vi "configure runtime data.vi"(4 "output dictionary":refnum<class "data dictionary.lvclass">, 6 "input dictionary":refnum<class "data dictionary.lvclass">, 8 "error in":errorcluster, 10 "Slave Info List":T4(array[cluster]), 11 "Profibus Module configuration in":refnum<class "Profibus Module configuration.lvclass">) -> (0 "error out":errorcluster, 2 "inputs":T1[](array[typedef]), 3 "outputs":T1[](array[typedef]))   [LabVIEW 2013, in "Profibus Module runtime.lvclass"]
uses:
  Profibus Module runtime.lvclass
  configuration/Profibus Module configuration.lvclass
  profibus slave configuration.ctl
  profibus mapping configuration.ctl
  <vilib>/NI/Tag Bus/tag/Data Type.ctl
  <vilib>/NI/Tag Bus/dictionary/data dictionary.lvclass
  configuration/Profibus Module configuration.lvclass/Profibus Module configuration.ctl
  channel/Profibus channel.lvclass/Profibus channel.ctl
  <vilib>/NI/Tag Bus Module Framework/channel/TBM channel.lvclass/TBM channel.ctl
  <vilib>/NI/Tag Bus/tag/tag descriptor.lvclass/tag descriptor.ctl
  <vilib>/NI/Tag Bus/tag/tag descriptor.lvclass
  <vilib>/NI/Tag Bus Module Framework/channel/TBM channel.lvclass
  channel/Profibus channel.lvclass
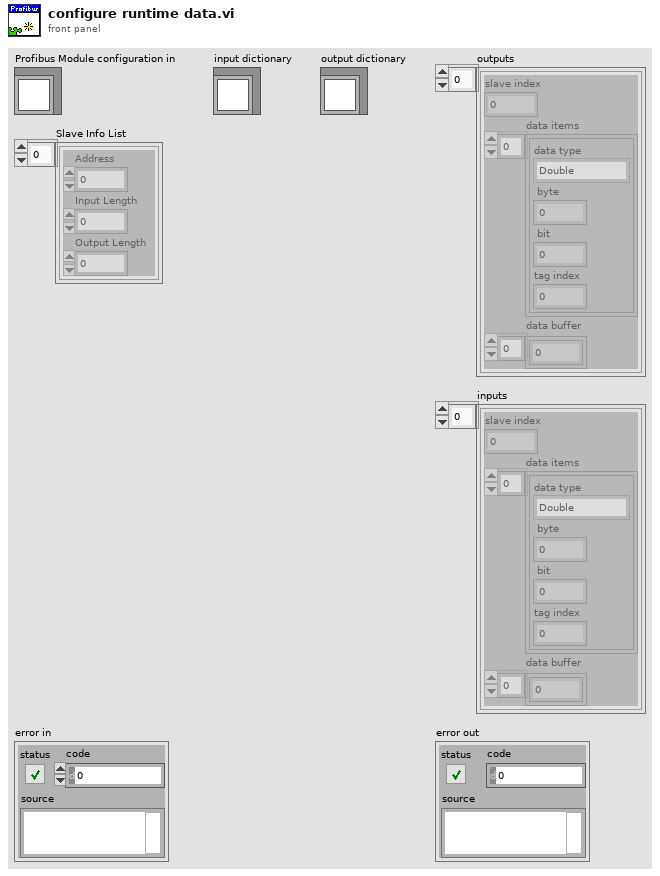
[diagram p1: front panel]
types:
  T1 = typedef "Profibus Module runtime.lvclass/profibus slave configuration.ctl" = cluster{"slave index":i8, "data items":T2[], "data buffer":u8[]}
  T2 = typedef "Profibus Module runtime.lvclass/profibus mapping configuration.ctl" = cluster{"data type":T3, " byte":i32, " bit":i32, "tag index":i32}
  T3 = typedef "tag bus.lvlib/tag descriptor.lvclass/Data Type.ctl" = enum16{"Double", "Single", "I64", "I32", "I16", "I8", "U64", "U32", "U16", "U8", "Boolean", "String", "Array of Double", "Array of Single", "Array of I64", "Array of I32", "Array of I16", "Array of I8", "Array of U64", "Array of U32", "Array of U16", "Array of U8", "Array of Boolean", "Array of String"}
  T4 = cluster{"Address":i8, "Input Length":u8, "Output Length":u8}[]
  T5 = typedef "TBM channel.lvclass/channel classification.ctl" = enum16{"input data", "output data", "processing parameter", "processing result"}
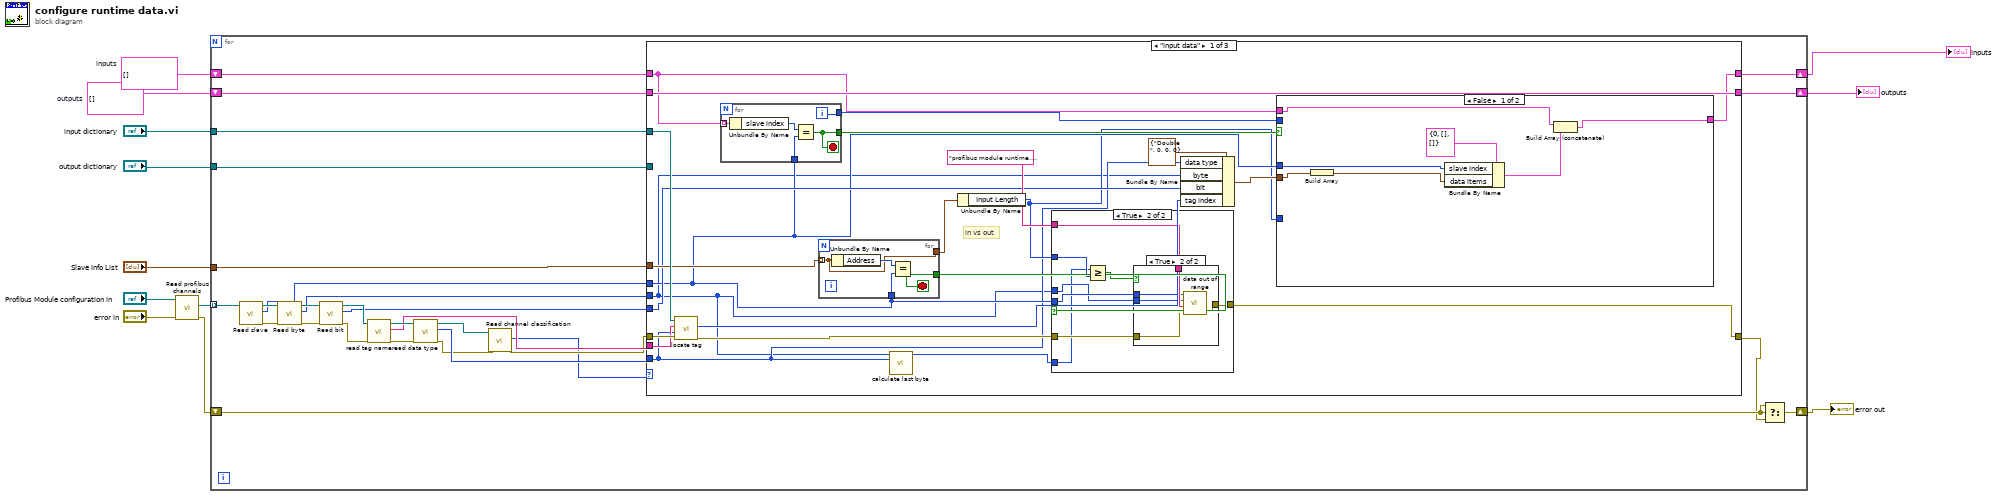
[diagram p0: block diagram]
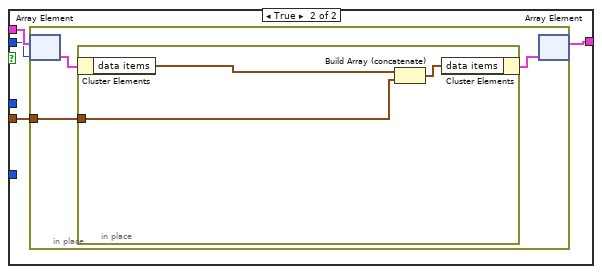
[diagram p2: hidden frame]
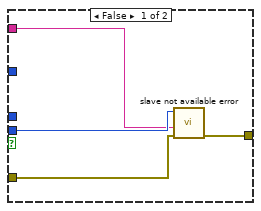
[diagram p3: hidden frame]
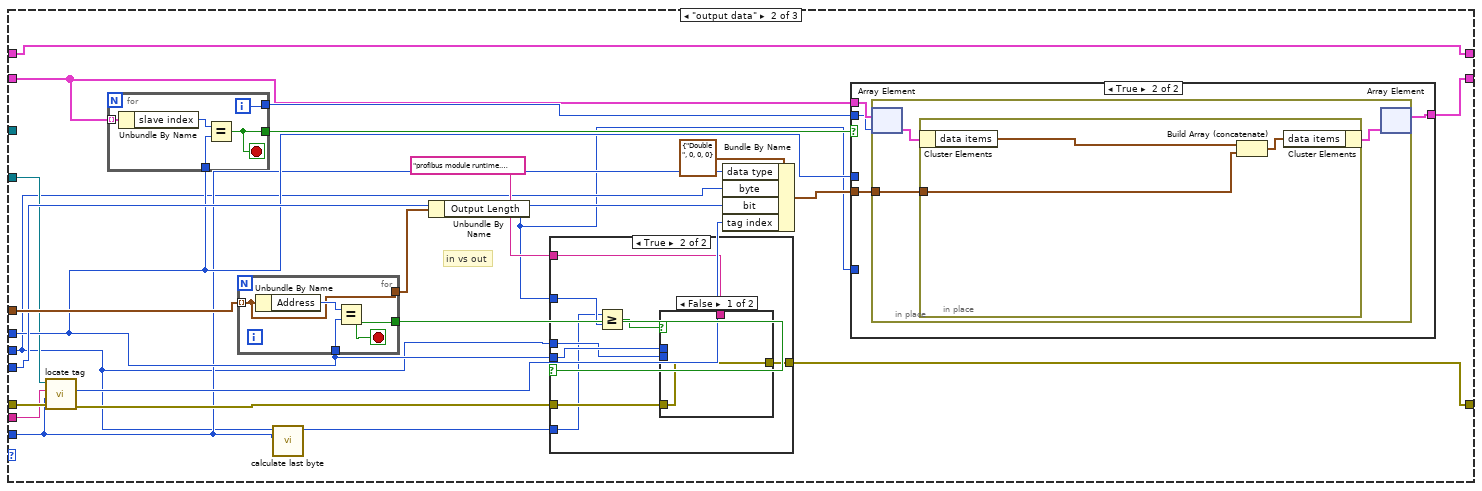
[diagram p5: hidden frame]
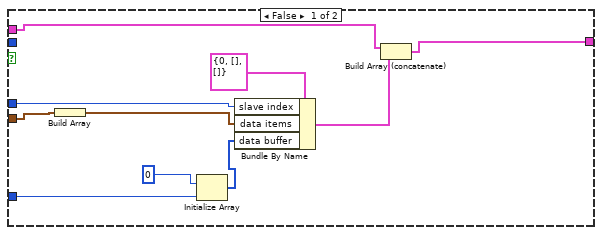
[diagram p6: hidden frame]
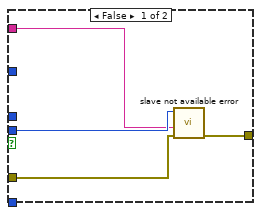
[diagram p7: hidden frame]
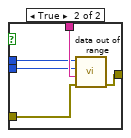
[diagram p8: hidden frame]
diagram:
  w6 = T1[] []  # outputs
  w7 = T1[] []  # inputs
  n1 = call "Read profibus channels.vi"("error in"="error in", "Profibus Module configuration in"="Profibus Module configuration in") -> ("error out"=w10:errorcluster, "channels"=w8:refnum<class "Profibus channel.lvclass">[])  [unwired: 7 in, 1 out]
  n2 = for {
    shift-right: [w39] -> w9
    shift-left: w10 -> [w40]
    tunnel: w8 -> [w22] mode=indexing
    shift-right: [w35] -> w1
    shift-left: w7 -> [w34]
    shift-right: [w33] -> w5
    shift-left: w6 -> [w32]
    tunnel: "Slave Info List" -> [w36]
    tunnel: "input dictionary" -> [w38]
    tunnel: "output dictionary" -> [w37]
    n3 = call "Read slave.vi"("Profibus channel in"=w22) -> ("error out"=w19:errorcluster, "slave"=w15:i8, "Profibus channel out"=w20:refnum<class "Profibus channel.lvclass">)  [unwired: 8 in]
    n4 = call "Read byte.vi"("error in"=w19, "Profibus channel in"=w20) -> ("error out"=w18:errorcluster, "byte"=w14:i32, "Profibus channel out"=w21:refnum<class "Profibus channel.lvclass">)  [unwired: 7 in]
    n5 = call "Read bit.vi"("error in"=w18, "Profibus channel in"=w21) -> ("error out"=w17:errorcluster, "bit"=w13:i32, "Profibus channel out"=w16:refnum<class "Profibus channel.lvclass">)  [unwired: 7 in]
    n6 = call <vilib>:"read tag name.vi"("error in"=w17, "system tag in"=w16) -> ("error out"=w27:errorcluster, "name"=w28:string, "system tag out"=w30:refnum<class "Profibus channel.lvclass">)  [unwired: 7 in]
    n7 = call <vilib>:"read data type.vi"("error in"=w27, "system tag in"=w30) -> ("error out"=w25:errorcluster, "data type"=w26:T3, "system tag out"=w29:refnum<class "Profibus channel.lvclass">)  [unwired: 7 in]
    n8 = call <vilib>:"Read channel classification.vi"("error in"=w25, "channel in"=w29) -> ("error out"=w24:errorcluster, "channel classification"=w23:T5)  [unwired: 7 in, 1 out]
    n9 = case shown="\"input data\"" w23 {
      tunnel: w24 -> [w62 w130 w178]
      tunnel: w26 -> [w43 w111 _]
      tunnel: w38 -> [w60 _ _]
      tunnel: w37 -> [_ w115 _]
      tunnel: w36 -> [w59 w128 _]
      tunnel: [w50 w112 w180] -> w35
      tunnel: w34 -> [w51 w112 w180]
      tunnel: [w63 w113 w179] -> w33
      tunnel: w32 -> [w63 w114 w179]
      tunnel: [w57 w126 w178] -> w31
      tunnel: w15 -> [w45 w116 _]
      tunnel: w14 -> [w42 w110 _]
      tunnel: w13 -> [w47 w118 _]
      tunnel: w28 -> [w61 w129 _]
      frame "input data" {
        # "in vs out"
        n10 = call <vilib>:"locate tag.vi"("error in"=w62, "data type"=w43, "name"=w61, "data dictionary in"=w60) -> ("error out"=w58:errorcluster, "index"=w46:i32)  [unwired: 5 in, 1 out]
        n11 = for {
          tunnel: w51 -> [w107] mode=indexing
          tunnel: w45 -> [w105]
          tunnel: [w104] -> w53
          tunnel: [w103] -> w52
          i -> [w103]
          stop <- w104 stop-if-true
          n12 = Unbundle By Name(w107) -> ("slave index"=w106:i8)
          n13 = Equal?(x=w106, y=w105) -> (x = y?=w104:bool)
        }
        n14 = for {
          tunnel: w59 -> [w99] mode=indexing
          tunnel: w45 -> [w101]
          tunnel: [w100] -> w56
          tunnel: [w99] -> w55
          stop <- w100 stop-if-true
          n15 = Unbundle By Name(w99) -> ("Address"=w102:i8)
          n16 = Equal?(x=w102, y=w101) -> (x = y?=w100:bool)
        }
        n17 = call "calculate last byte.vi"("type"=w43, "byte in"=w42) -> ("last byte"=w41:i32)  [unwired: 9 in]
        n18 = Unbundle By Name(w55) -> ("Input Length"=w44:u8)
        n19 = case shown="True" w56 {
          tunnel: w58 -> [w84 w91]
          tunnel: [w83 w92] -> w57
          tunnel: w45 -> [w82 w88]
          tunnel: w44 -> [_ w89]
          tunnel: w42 -> [_ w87]
          tunnel: "profibus module runtime.lvclass>>init.vi>>configure runtime data.vi" ("source") -> [w81 w90]
          tunnel: w41 -> [_ w85]
          frame False {
            n20 = call "slave not available error.vi"("error in"=w84, "source"=w81, "slave"=w82) -> ("error out"=w83:errorcluster)  [unwired: 8 in]
          }
          frame True {
            n21 = Greater Or Equal?(x=w85, y=w89) -> (x >= y?=w86:bool)
            n22 = case shown="True" w86 {
              tunnel: [w93 w98] -> w92
              tunnel: w91 -> [w93 w97]
              tunnel: w90 -> [_ w96]
              tunnel: w88 -> [_ w95]
              tunnel: w87 -> [_ w94]
              frame False {
              }
              frame True {
                n23 = call "data out of range.vi"("error in"=w97, "source"=w96, "byte"=w94, "slave"=w95) -> ("error out"=w98:errorcluster)  [unwired: 7 in]
              }
            }
          }
        }
        n24 = Bundle By Name(cluster=T2 {"data type"=enum."Double", " byte"=0, " bit"=0, "tag index"=0} ("data items"), "data type"=w43, "byte"=w42, "bit"=w47, "tag index"=w46) -> (w48:T2)
        n25 = case shown="False" w53 {
          tunnel: w52 -> [_ w73]
          tunnel: w51 -> [w70 w74]
          tunnel: [w69 w72] -> w50
          tunnel: w48 -> [w66 w71]
          tunnel: w45 -> [w64 _]
          tunnel: w44 -> [_ _]
          frame False {
            n26 = Build Array(w66) -> (w65:T2[])
            n27 = Bundle By Name(cluster=T1 {"slave index"=0, "data items"=[], "data buffer"=[]} ("slave configuration"), "slave index"=w64, "data items"=w65) -> (w67:T1)
            n28 = Build Array (concatenate)(w70, w67) -> (w69:T1[])
          }
          frame True {
            n29 = in-place {
              in-place-border: w71 -> [w75]
              n30 = in-place-array #1(w74, w73) -> (w77:T1)
              n31 = in-place {
                in-place-border: w75 -> [w78]
                n32 = in-place-cluster #2(w77) -> ("data items"=w80:T2[])
                n33 = Build Array (concatenate)(w80, w78) -> (w79:T2[])
                n34 = in-place-cluster #2("data items"=w79) -> (w76:T1)
              }
              n35 = in-place-array #1(w76) -> (w72:T1[])  [unwired: 1 out]
            }
          }
        }
      }
      frame "output data" {
        # "in vs out"
        n36 = call <vilib>:"locate tag.vi"("error in"=w130, "data type"=w111, "name"=w129, "data dictionary in"=w115) -> ("error out"=w127:errorcluster, "index"=w117:i32)  [unwired: 5 in, 1 out]
        n37 = for {
          tunnel: w114 -> [w177] mode=indexing
          tunnel: w116 -> [w175]
          tunnel: [w174] -> w122
          tunnel: [w173] -> w121
          i -> [w173]
          stop <- w174 stop-if-true
          n38 = Unbundle By Name(w177) -> ("slave index"=w176:i8)
          n39 = Equal?(x=w176, y=w175) -> (x = y?=w174:bool)
        }
        n40 = for {
          tunnel: w128 -> [w169] mode=indexing
          tunnel: w116 -> [w171]
          tunnel: [w170] -> w125
          tunnel: [w169] -> w124
          stop <- w170 stop-if-true
          n41 = Unbundle By Name(w169) -> ("Address"=w172:i8)
          n42 = Equal?(x=w172, y=w171) -> (x = y?=w170:bool)
        }
        n43 = call "calculate last byte.vi"("type"=w111, "byte in"=w110) -> ("last byte"=w109:i32)  [unwired: 9 in]
        n44 = Unbundle By Name(w124) -> ("Output Length"=w108:u8)
        n45 = case shown="True" w125 {
          tunnel: w127 -> [w154 w161]
          tunnel: [w153 w162] -> w126
          tunnel: w116 -> [w152 w158]
          tunnel: w108 -> [_ w159]
          tunnel: w110 -> [_ w156]
          tunnel: "profibus module runtime.lvclass>>init.vi>>configure runtime data.vi" ("source") -> [w151 w160]
          tunnel: w109 -> [_ w155]
          frame False {
            n46 = call "slave not available error.vi"("error in"=w154, "source"=w151, "slave"=w152) -> ("error out"=w153:errorcluster)  [unwired: 8 in]
          }
          frame True {
            n47 = Greater Or Equal?(x=w155, y=w159) -> (x >= y?=w157:bool)
            n48 = case shown="False" w157 {
              tunnel: [w163 w168] -> w162
              tunnel: w161 -> [w163 w167]
              tunnel: w160 -> [_ w166]
              tunnel: w158 -> [_ w165]
              tunnel: w156 -> [_ w164]
              frame False {
              }
              frame True {
                n49 = call "data out of range.vi"("error in"=w167, "source"=w166, "byte"=w164, "slave"=w165) -> ("error out"=w168:errorcluster)  [unwired: 7 in]
              }
            }
          }
        }
        n50 = Bundle By Name(cluster=T2 {"data type"=enum."Double", " byte"=0, " bit"=0, "tag index"=0} ("data items"), "data type"=w111, "byte"=w110, "bit"=w118, "tag index"=w117) -> (w119:T2)
        n51 = case shown="True" w122 {
          tunnel: w121 -> [_ w143]
          tunnel: w114 -> [w140 w144]
          tunnel: [w139 w142] -> w113
          tunnel: w119 -> [w136 w141]
          tunnel: w116 -> [w134 _]
          tunnel: w108 -> [w132 _]
          frame False {
            n52 = Build Array(w136) -> (w135:T2[])
            n53 = Initialize Array(u8 0 ("Numeric"), w132) -> (w131:u8[])
            n54 = Bundle By Name(cluster=T1 {"slave index"=0, "data items"=[], "data buffer"=[]} ("slave configuration"), "slave index"=w134, "data items"=w135, "data buffer"=w131) -> (w137:T1)
            n55 = Build Array (concatenate)(w140, w137) -> (w139:T1[])
          }
          frame True {
            n56 = in-place {
              in-place-border: w141 -> [w145]
              n57 = in-place-array #3(w144, w143) -> (w147:T1)
              n58 = in-place {
                in-place-border: w145 -> [w148]
                n59 = in-place-cluster #4(w147) -> ("data items"=w150:T2[])
                n60 = Build Array (concatenate)(w150, w148) -> (w149:T2[])
                n61 = in-place-cluster #4("data items"=w149) -> (w146:T1)
              }
              n62 = in-place-array #3(w146) -> (w142:T1[])  [unwired: 1 out]
            }
          }
        }
      }
      frame Default {
      }
    }
    n63 = Select(t=w40, s=w40, f=w31) -> (s? t:f=w39:errorcluster)
  }
  "error out" <- w9
  "inputs" <- w1
  "outputs" <- w5
